vi "Calibration tool box main GUI update.vi"(7 "Actions":T3(ring), 8 "error in (no error)":errorcluster, 11 "Calibration GUI parameters":T2) -> (0 "error out":errorcluster, 2 "Updated frame size":T1=200 items=["100X100"=100, "128X128"=128, "200X200"=200, "256X256"=256, "512X512"=512, "1024x1024"=1024, "2048x2048"=2048], 3 "Current Objective":string)   [LabVIEW 2020]
uses:
  TypeDefs/Calibration GUI parameter refs.ctl
  Typedefs/Objective selector control enum.ctl
  Typedefs/Frame Size.ctl
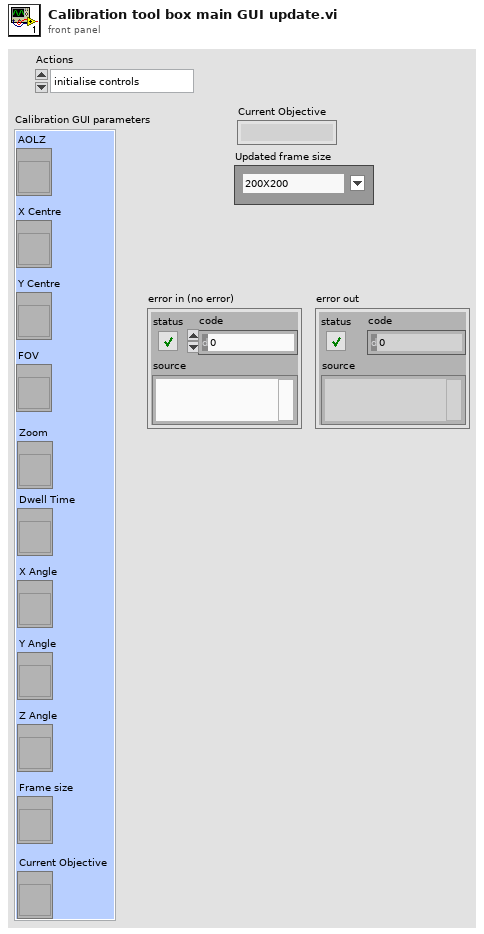
[diagram p1: front panel]
types:
  T1 = typedef "Frame Size.ctl" = u16
  T2 = typedef "Calibration GUI parameter refs.ctl" = cluster{"AOLZ":refnum<vi>, "X Centre":refnum<vi>, "Y Centre":refnum<vi>, "FOV":refnum<vi>, "Dwell Time":refnum<vi>, "X Angle":refnum<vi>, "Y Angle":refnum<vi>, "Z Angle":refnum<vi>, "Frame size":refnum<vi>, "Current Objective":refnum<vi>, "Zoom":refnum<vi>}
  T3 = enum16{"initialise controls", "Update to main GUI", "Update to calib toolbox "}
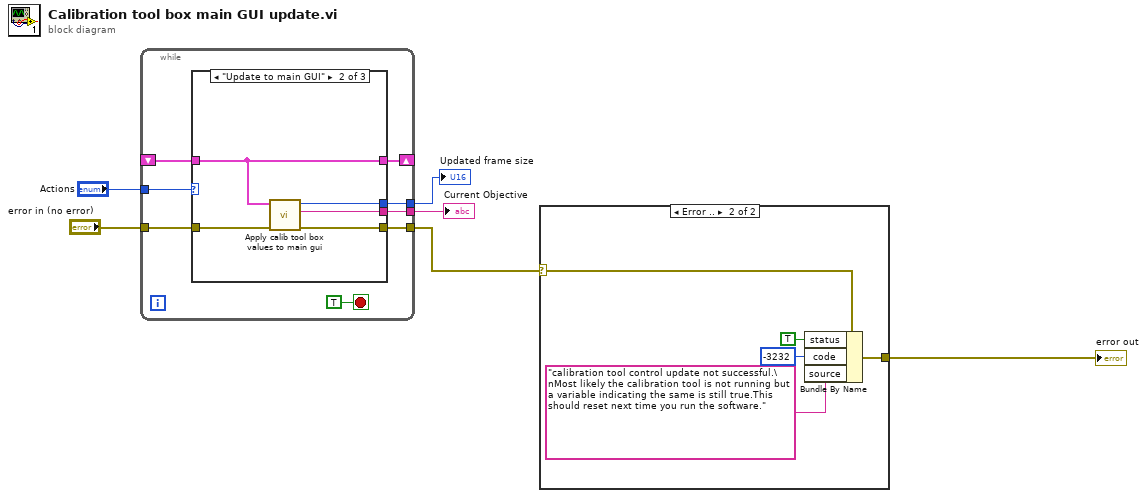
[diagram p0: block diagram]
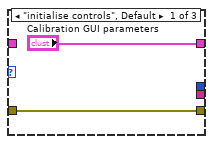
[diagram p3: hidden frame]
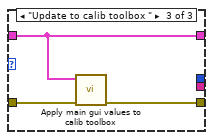
[diagram p4: hidden frame]
diagram:
  n1 = while {
    tunnel: "Actions" -> [w14]
    shift-right: [w13] -> _
    shift-left: _ -> [w12]
    tunnel: "error in (no error)" -> [w10]
    tunnel: [w9] -> w2
    tunnel: [w8] -> w4
    tunnel: [w7] -> w3
    stop <- TRUE stop-if-true
    n2 = case shown="\"Update to main GUI\"" w14 {
      tunnel: ["Calibration GUI parameters" w21 w24] -> w13
      tunnel: w12 -> [_ w21 w24]
      tunnel: w10 -> [w15 w20 w23]
      tunnel: [w15 w19 w22] -> w9
      tunnel: [_ w18 _] -> w8
      tunnel: [_ w17 _] -> w7
      frame "initialise controls", Default {
      }
      frame "Update to main GUI" {
        n3 = call "Apply calib tool box values to main gui.vi"("error in (no error)"=w20, "Calibration GUI parameters in"=w21) -> ("error out"=w19:errorcluster, "Current Objective"=w17:string, "Updated frame size"=w18:T1)  [unwired: 7 in]
      }
      frame "Update to calib toolbox " {
        n4 = call "Apply main gui values to calib toolbox.vi"("error in (no error)"=w23, "Calibration GUI parameters in"=w24) -> ("error out"=w22:errorcluster)  [unwired: 9 in]
      }
    }
  }
  "Updated frame size" <- w4
  "Current Objective" <- w3
  n5 = case shown="Error .." w2 {
    selector: w2 -> [w25 w30]
    tunnel: [w25 w29] -> w1
    frame No Error {
    }
    frame Error {
      n6 = Bundle By Name(cluster=w30, "status"=TRUE, "code"=-3232, "source"="calibration tool control update not successful.\nMost likely the calibration tool is not running but a variable indicating the same is still true.This should reset next time you run the software.") -> (w29:errorcluster)
    }
  }
  "error out" <- w1
